vi "fpga_Filter Constant (P Class).vi"() -> (0 "Total Delay":u8=15, 1 "Start":fxp<+/-,4,4>=1.0, 2 "LP2 delay":u8=15, 3 "LP1 delay":u8=3)   [LabVIEW 2013, in "NI_EP_PMU_FPGA.lvlib"]
uses:
  <vilib>/addons/Electrical Power/PMU/NI_EP_PMU_FPGA.lvlib
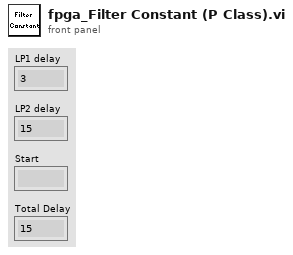
[diagram p1: front panel]
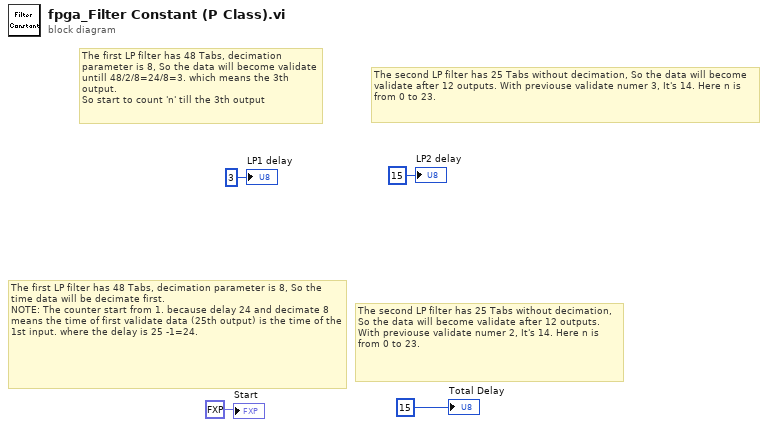
[diagram p0: block diagram]
diagram:
  # "The first LP filter has 48 Tabs, decimation parameter is 8, So the data will become validate untill 48/2/8=24/8=3. which means the 3th output.\nSo start to count 'n' till the 3th output"
  # "The second LP filter has 25 Tabs without decimation, So the data will become validate after 12 outputs. With previouse validate numer 3, It's 14. Here n is from 0 to 23."
  # "The second LP filter has 25 Tabs without decimation, So the data will become validate after 12 outputs. With previouse validate numer 2, It's 14. Here n is from 0 to 23."
  # "The first LP filter has 48 Tabs, decimation parameter is 8, So the time data will be decimate first.\nNOTE: The counter start from 1. because delay 24 and decimate 8 means the time of first validate data (25th output) is the time of the 1st input. where the delay is 25 -1=24."
  "Start" <- fxp<+/-,4,4> 1.0 ("Start")
  "Total Delay" <- u8 15 ("Total Delay")
  "LP1 delay" <- u8 3 ("n-1[0..15]")
  "LP2 delay" <- u8 15 ("n-1[0..23]")
